vi "initialize_projector.vi"(3 "BlueCurrent":u8=130, 4 "RedBluePatternRepeat":i32=1, 5 "GreenCurrent":u8=135, 6 "Green Only":bool, 7 "RedCurrent":u8=104, 8 "error in":errorcluster, 9 "blue exp_time_us":i32=8215, 10 "red exp_time_us":i32=8215, 11 "green exp_time_us":i32=235) -> (0 "error out":errorcluster)   [LabVIEW 2019]
panel:
  out "numLutEntries":i32
  out "Sequence Validation Results":bool[](array[boolean])
  # "Exposure/Period out of range"
  # "Pattern Number out of range"
  # "continuous TriggerOut1 request or overlapping black sectors"
  # "post vector was not inserted prior to external triggered vector"
  # "frame period or exposure difference is less than 230usec"
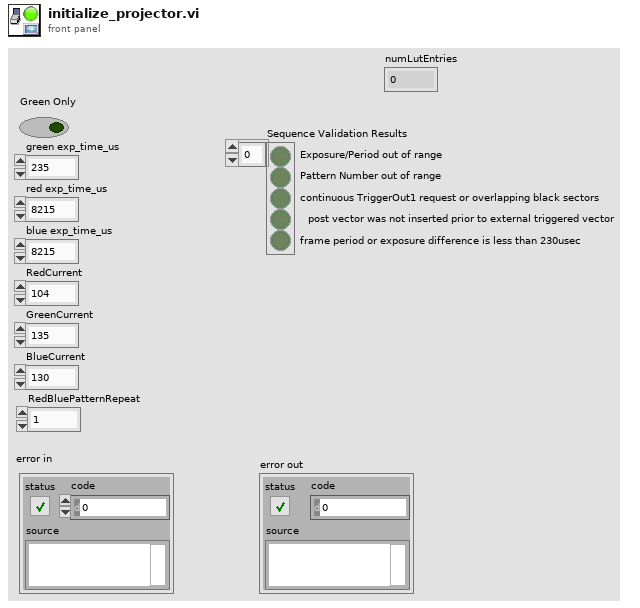
[diagram p1: front panel]
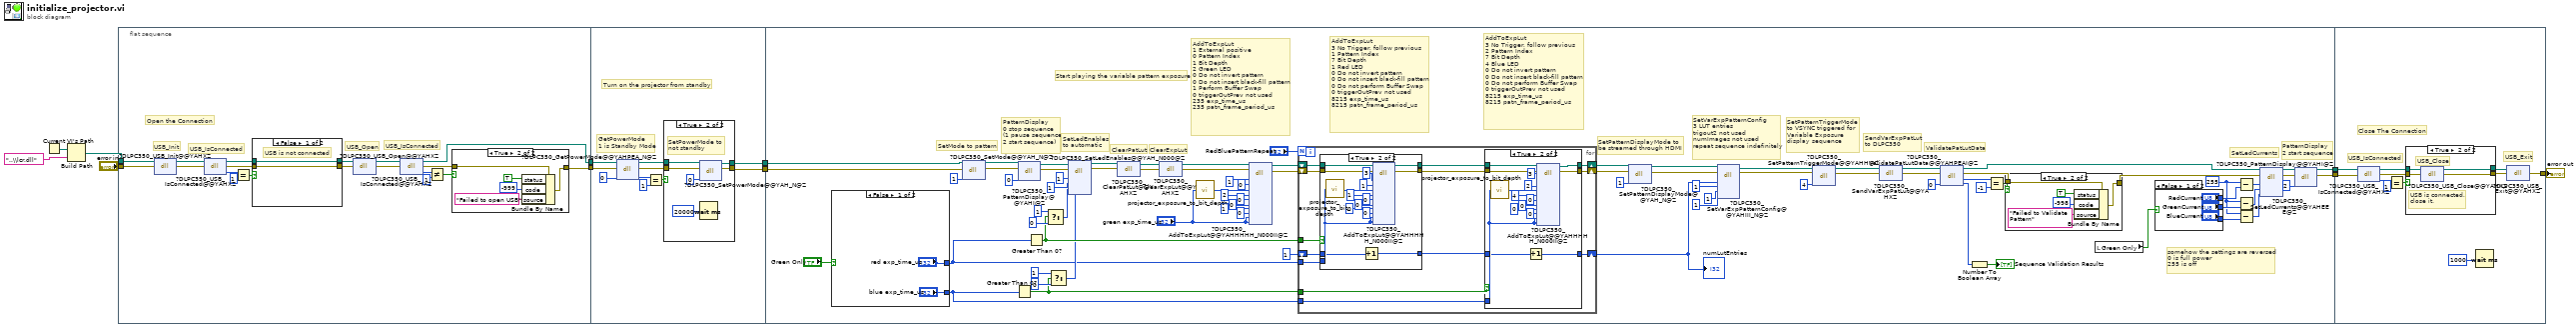
[diagram p0: block diagram]
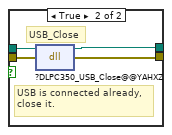
[diagram p3: hidden frame]
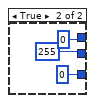
[diagram p7: hidden frame]
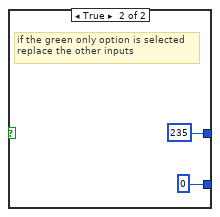
[diagram p8: hidden frame]
diagram:
  n1 = Current VI's Path() -> (path=w6:path)
  n2 = Build Path(base path=w6, name or relative path="..\\lcr.dll") -> (appended path=w4:path)
  n3 = flat-sequence {
    tunnel: [w20] -> w9
    tunnel: "error in" -> [w19]
    tunnel: w4 -> [w18]
    tunnel: [w13] -> w3
    tunnel: w9 -> [w50]
    tunnel: [w52] -> w8
    tunnel: w3 -> [w45]
    tunnel: [w43] -> w2
    tunnel: [w94] -> w10
    tunnel: w8 -> [w108]
    tunnel: w2 -> [w107]
    tunnel: [w92] -> w1
    tunnel: [w209] -> w11
    tunnel: w10 -> [w208]
    tunnel: w1 -> [w207]
    frame #0 {
      # "Open the Connection"
      # "USB_IsConnected"
      # "USB_Open"
      # "USB_IsConnected"
      # "USB_Init"
      n4 = dll-call lib="C:/Users/mochil/Dropbox/LeiferShaevitz/Github/ProjectAPI/LabviewVIs/lcr.dll" fn="?DLPC350_USB_Init@@YAHXZ"(path in=w18, error in=w19) -> (path out=w17:path, error out=w30:errorcluster)  [unwired: 2 in]
      n5 = dll-call lib="C:/Users/mochil/Dropbox/LeiferShaevitz/Github/ProjectAPI/LabviewVIs/lcr.dll" fn="?DLPC350_USB_IsConnected@@YAHXZ"(path in=w17, error in=w30) -> (path out=w16:path, error out=w27:errorcluster, "return type"=w22:i32)  [unwired: 1 in]
      n6 = Equal?(x=w22, y=1) -> (x = y?=w28:bool)
      n7 = case shown="False" w28 {
        tunnel: w27 -> [w38 w42]
        tunnel: [w38 w41] -> w29
        tunnel: w16 -> [w37 w40]
        tunnel: [w37 w39] -> w15
        frame False {
          # "USB is not connected"
        }
        frame True {
          # "USB_Close"
          # "USB is connected already,\nclose it."
          n8 = dll-call lib="C:/Users/mochil/Dropbox/LeiferShaevitz/Github/ProjectAPI/LabviewVIs/lcr.dll" fn="?DLPC350_USB_Close@@YAHXZ"(path in=w40, error in=w42) -> (path out=w39:path, error out=w41:errorcluster)  [unwired: 2 in]
        }
      }
      n9 = dll-call lib="C:/Users/mochil/Dropbox/LeiferShaevitz/Github/ProjectAPI/LabviewVIs/lcr.dll" fn="?DLPC350_USB_Open@@YAHXZ"(path in=w15, error in=w29) -> (path out=w14:path, error out=w26:errorcluster)  [unwired: 2 in]
      n10 = dll-call lib="C:/Users/mochil/Dropbox/LeiferShaevitz/Github/ProjectAPI/LabviewVIs/lcr.dll" fn="?DLPC350_USB_IsConnected@@YAHXZ"(path in=w14, error in=w26) -> (path out=w13:path, error out=w23:errorcluster, "return type"=w12:i32)  [unwired: 1 in]
      n11 = Not Equal?(x=w12, y=1) -> (x != y?=w24:bool)
      n12 = case shown="True" w24 {
        tunnel: w23 -> [w31 w33]
        tunnel: [w31 w32] -> w20
        frame False {
        }
        frame True {
          n13 = Bundle By Name(cluster=w33, "status"=TRUE, "code"=-999, "source"="Failed to open USB") -> (w32:errorcluster)
        }
      }
    }
    frame #1 {
      # "Turn on the projector from standby"
      # "GetPowerMode\n1 is Standby Mode"
      n14 = dll-call lib="C:/Users/mochil/Dropbox/LeiferShaevitz/Github/ProjectAPI/LabviewVIs/lcr.dll" fn="?DLPC350_GetPowerMode@@YAHPEA_N@Z"(path in=w45, error in=w50, "pStandby"=0) -> (path out=w44:path, error out=w46:errorcluster, "pStandby"=w49:i32)  [unwired: 2 in]
      n15 = Equal?(x=w49, y=1) -> (x = y?=w47:bool)
      n16 = case shown="True" w47 {
        tunnel: [w54 w59] -> w52
        tunnel: w46 -> [w54 w58]
        tunnel: w44 -> [w53 w56]
        tunnel: [w53 w55] -> w43
        frame False {
        }
        frame True {
          # "SetPowerMode to\nnot standby"
          n17 = dll-call lib="C:/Users/mochil/Dropbox/LeiferShaevitz/Github/ProjectAPI/LabviewVIs/lcr.dll" fn="?DLPC350_SetPowerMode@@YAH_N@Z"(path in=w56, error in=w58, "Standby"=0) -> (path out=w55:path, error out=w59:errorcluster)  [unwired: 3 in]
          n18 = Wait (ms)(milliseconds to wait=20000) -> ()  [unwired: 1 out]
        }
      }
    }
    frame #2 {
      w87 = u8 255 ("RedCurrent")
      # "ClearExpLut"
      # "somehow the settings are reversed\n0 is full power\n255 is off"
      # "PatternDisplay\n2 start sequence"
      # "SetLedCurrents"
      # "Start playing the variable pattern exposure"
      # "ValidatePatLutData"
      # "SetPatternTriggerMode\nto VSYNC triggered for \nVariable Exposure \ndisplay sequence"
      # "SetPatternDisplayMode to\nbe streamed through HDMI"
      # "AddToExpLut\n3 No Trigger, follow previous\n2 Pattern Index\n7 Bit Depth\n4 Blue LED\n0 Do not invert pattern\n0 Do not insert black-fill pattern\n0 Do not perform Buffer Swap\n0 triggerOutPrev not used\n8215 exp_time_us\n8215 patn_frame_period_us"
      # "AddToExpLut\n3 No Trigger, follow previous\n1 Pattern Index\n7 Bit Depth\n1 Red LED\n0 Do not invert pattern\n0 Do not insert black-fill pattern\n0 Do not perform Buffer Swap\n0 triggerOutPrev not used\n8215 exp_time_us\n8215 patn_frame_period_us"
      # "AddToExpLut\n1 External positive\n0 Pattern Index\n1 Bit Depth\n2 Green LED\n0 Do not invert pattern\n0 Do not insert black-fill pattern\n1 Perform Buffer Swap\n0 triggerOutPrev not used\n235 exp_time_us\n235 patn_frame_period_us"
      # "SendVarExpPatLut\nto DLPC350"
      # "SetVarExpPatternConfig\n3 LUT entries\ntrigout2 not used\nnumImages not used\nrepeat sequence indefinitely"
      # "ClearPatLut"
      # "PatternDisplay\n0 stop sequence\n(1 pause sequence\n2 start sequence)"
      # "SetLedEnables \nto automatic"
      # "SetMode to pattern"
      n19 = case shown="False" "Green Only" {
        tunnel: ["blue exp_time_us" 0 ("blue exp_time_us")] -> w67
        tunnel: ["red exp_time_us" 235 ("red exp_time_us")] -> w66
        frame False {
        }
        frame True {
          # "if the green only option is selected\nreplace the other inputs"
        }
      }
      n20 = dll-call lib="C:/Users/mochil/Dropbox/LeiferShaevitz/Github/ProjectAPI/LabviewVIs/lcr.dll" fn="?DLPC350_SetMode@@YAH_N@Z"(path in=w107, error in=w108, "SLmode"=1) -> (path out=w106:path, error out=w135:errorcluster)  [unwired: 3 in]
      n21 = Greater Than 0?(x=w67) -> (x > 0?=w72:bool)
      n22 = dll-call lib="C:/Users/mochil/Dropbox/LeiferShaevitz/Github/ProjectAPI/LabviewVIs/lcr.dll" fn="?DLPC350_PatternDisplay@@YAHI@Z"(path in=w106, error in=w135, "Action"=0) -> (path out=w105:path, error out=w134:errorcluster)  [unwired: 3 in]
      n23 = Greater Than 0?(x=w66) -> (x > 0?=w77:bool)
      n24 = Select(t=1 ("green"), s=w77, f=0) -> (s? t:f=w76:i32)
      n25 = Select(t=1 ("green"), s=w72, f=0) -> (s? t:f=w73:i32)
      n26 = dll-call lib="C:/Users/mochil/Dropbox/LeiferShaevitz/Github/ProjectAPI/LabviewVIs/lcr.dll" fn="?DLPC350_SetLedEnables@@YAH_N000@Z"(path in=w105, error in=w134, "seqCtrl"=1, "red"=w76, "green"=1, "blue"=w73) -> (path out=w104:path, error out=w133:errorcluster)  [unwired: 6 in]
      n27 = dll-call lib="C:/Users/mochil/Dropbox/LeiferShaevitz/Github/ProjectAPI/LabviewVIs/lcr.dll" fn="?DLPC350_ClearPatLut@@YAHXZ"(path in=w104, error in=w133) -> (path out=w70:path, error out=w71:errorcluster)  [unwired: 2 in]
      n28 = dll-call lib="C:/github/ProjectAPI/LabviewVIs/lcr.dll" fn="?DLPC350_ClearExpLut@@YAHXZ"(path in=w70, error in=w71) -> (path out=w69:path, error out=w68:errorcluster)  [unwired: 2 in]
      n29 = call "projector_exposure_to_bit_depth.vi"("exp_time_us"="green exp_time_us") -> ("BitDepth"=w83:i32)
      n30 = dll-call lib="C:/Users/mochil/Dropbox/LeiferShaevitz/Github/ProjectAPI/LabviewVIs/lcr.dll" fn="?DLPC350_AddToExpLut@@YAHHHHH_N000II@Z"(path in=w69, error in=w68, "TrigType"=1, "PatNum"=0, "BitDepth"=w83, "LEDSelect"=2, "InvertPat"=0, "InsertBlack"=0, "BufSwap"=1, "trigOutPrev"=0, "exp_time_us"="green exp_time_us", "ptn_frame_period_us"="green exp_time_us") -> (path out=w82:path, error out=w81:errorcluster)  [unwired: 12 in]
      n31 = for {
        N: "RedBluePatternRepeat" -> [_]
        tunnel: w77 -> [w144]
        tunnel: w72 -> [w143]
        tunnel: w67 -> [w142]
        tunnel: w66 -> [w141]
        shift-right: [w151] -> w103
        shift-left: w82 -> [w146]
        shift-right: [w139] -> w121
        shift-left: w81 -> [w145]
        shift-right: [w140] -> w62
        shift-left: 1 ("numLutEntries") -> [w150]
        n32 = case shown="True" w144 {
          tunnel: w145 -> [w153 w163]
          tunnel: [w153 w162] -> w148
          tunnel: w146 -> [w154 w161]
          tunnel: [w154 w160] -> w147
          tunnel: w141 -> [_ w159]
          tunnel: w150 -> [w152 w156]
          tunnel: [w152 w157] -> w149
          frame False {
          }
          frame True {
            n33 = call "projector_exposure_to_bit_depth.vi"("exp_time_us"=w159) -> ("BitDepth"=w158:i32)
            n34 = Increment(x=w156) -> (x+1=w157:i32)
            n35 = dll-call lib="C:/Users/mochil/Dropbox/LeiferShaevitz/Github/ProjectAPI/LabviewVIs/lcr.dll" fn="?DLPC350_AddToExpLut@@YAHHHHH_N000II@Z"(path in=w161, error in=w163, "TrigType"=3, "PatNum"=1, "BitDepth"=w158, "LEDSelect"=1, "InvertPat"=0, "InsertBlack"=0, "BufSwap"=0, "trigOutPrev"=0, "exp_time_us"=w159, "ptn_frame_period_us"=w159) -> (path out=w160:path, error out=w162:errorcluster)  [unwired: 12 in]
          }
        }
        n36 = case shown="True" w143 {
          tunnel: w148 -> [w171 w181]
          tunnel: [w171 w180] -> w139
          tunnel: w147 -> [w172 w179]
          tunnel: [w172 w178] -> w151
          tunnel: w142 -> [_ w177]
          tunnel: w149 -> [w170 w174]
          tunnel: [w170 w175] -> w140
          frame False {
          }
          frame True {
            n37 = call "projector_exposure_to_bit_depth.vi"("exp_time_us"=w177) -> ("BitDepth"=w176:i32)
            n38 = Increment(x=w174) -> (x+1=w175:i32)
            n39 = dll-call lib="C:/Users/mochil/Dropbox/LeiferShaevitz/Github/ProjectAPI/LabviewVIs/lcr.dll" fn="?DLPC350_AddToExpLut@@YAHHHHH_N000II@Z"(path in=w179, error in=w181, "TrigType"=3, "PatNum"=2, "BitDepth"=w176, "LEDSelect"=4, "InvertPat"=0, "InsertBlack"=0, "BufSwap"=0, "trigOutPrev"=0, "exp_time_us"=w177, "ptn_frame_period_us"=w177) -> (path out=w178:path, error out=w180:errorcluster)  [unwired: 12 in]
          }
        }
      }
      "numLutEntries" <- w62
      n40 = dll-call lib="C:/Users/mochil/Dropbox/LeiferShaevitz/Github/ProjectAPI/LabviewVIs/lcr.dll" fn="?DLPC350_SetPatternDisplayMode@@YAH_N@Z"(path in=w103, error in=w121, "external"=1) -> (path out=w102:path, error out=w120:errorcluster)  [unwired: 3 in]
      n41 = dll-call lib="C:/Users/mochil/Dropbox/LeiferShaevitz/Github/ProjectAPI/LabviewVIs/lcr.dll" fn="?DLPC350_SetVarExpPatternConfig@@YAHIII_N@Z"(path in=w102, error in=w120, "numLutEntries"=w62, "numPatsForTrigOut2"=1 ("repeat"), "numImages"=1 ("numPatsForTrigOut2"), "repeat"=1 ("numImages")) -> (path out=w101:path, error out=w118:errorcluster)  [unwired: 6 in]
      n42 = dll-call lib="C:/Users/mochil/Dropbox/LeiferShaevitz/Github/ProjectAPI/LabviewVIs/lcr.dll" fn="?DLPC350_SetPatternTriggerMode@@YAHH@Z"(path in=w101, error in=w118, "trigMode"=4) -> (path out=w100:path, error out=w117:errorcluster)  [unwired: 3 in]
      n43 = dll-call lib="C:/Users/mochil/Dropbox/LeiferShaevitz/Github/ProjectAPI/LabviewVIs/lcr.dll" fn="?DLPC350_SendVarExpPatLut@@YAHXZ"(path in=w100, error in=w117) -> (path out=w99:path, error out=w116:errorcluster)  [unwired: 2 in]
      n44 = dll-call lib="C:/Users/mochil/Dropbox/LeiferShaevitz/Github/ProjectAPI/LabviewVIs/lcr.dll" fn="?DLPC350_ValidatePatLutData@@YAHPEAI@Z"(path in=w99, error in=w116, "pStatus"=0) -> (path out=w97:path, error out=w109:errorcluster, "return type"=w112:i32, "pStatus"=w114:i32)  [unwired: 1 in]
      n45 = Number To Boolean Array(number=w114) -> (Boolean array=→"Sequence Validation Results":bool[])
      n46 = Equal?(x=w112, y=-1) -> (x = y?=w110:bool)
      n47 = case shown="True" w110 {
        tunnel: w109 -> [w198 w200]
        tunnel: [w198 w199] -> w96
        frame False {
        }
        frame True {
          n48 = Bundle By Name(cluster=w200, "status"=TRUE, "code"=-998, "source"="Failed to Validate Pattern") -> (w199:errorcluster)
        }
      }
      n49 = local read "Green Only"() -> (w64:bool)
      n50 = case shown="False" w64 {
        tunnel: ["RedCurrent" u8 0 ("RedCurrent")] -> w90
        tunnel: ["GreenCurrent" u8 255 ("GreenCurrent")] -> w89
        tunnel: ["BlueCurrent" u8 0 ("BlueCurrent")] -> w86
        frame False {
        }
        frame True {
        }
      }
      n51 = Subtract(x=w87, y=w90) -> (x-y=w91:u8)
      n52 = Subtract(x=w87, y=w89) -> (x-y=w88:u8)
      n53 = Subtract(x=w87, y=w86) -> (x-y=w85:u8)
      n54 = dll-call lib="C:/Users/mochil/Dropbox/LeiferShaevitz/Github/ProjectAPI/LabviewVIs/lcr.dll" fn="?DLPC350_SetLedCurrents@@YAHEEE@Z"(path in=w97, error in=w96, "RedCurrent"=w91, "GreenCurrent"=w88, "BlueCurrent"=w85) -> (path out=w93:path, error out=w95:errorcluster)  [unwired: 5 in]
      n55 = dll-call lib="C:/Users/mochil/Dropbox/LeiferShaevitz/Github/ProjectAPI/LabviewVIs/lcr.dll" fn="?DLPC350_PatternDisplay@@YAHI@Z"(path in=w93, error in=w95, "Action"=2) -> (path out=w92:path, error out=w94:errorcluster)  [unwired: 3 in]
    }
    frame #3 {
      # "Close The Connection"
      # "USB_Exit"
      # "USB_IsConnected"
      n56 = dll-call lib="C:/Users/mochil/Dropbox/LeiferShaevitz/Github/ProjectAPI/LabviewVIs/lcr.dll" fn="?DLPC350_USB_IsConnected@@YAHXZ"(path in=w207, error in=w208) -> (path out=w206:path, error out=w212:errorcluster, "return type"=w213:i32)  [unwired: 1 in]
      n57 = Equal?(x=w213, y=1) -> (x = y?=w211:bool)
      n58 = case shown="True" w211 {
        tunnel: w212 -> [w216 w220]
        tunnel: [w216 w219] -> w214
        tunnel: w206 -> [w215 w218]
        tunnel: [w215 w217] -> w205
        frame False {
          # "USB is not connected"
        }
        frame True {
          # "USB_Close"
          # "USB is connected,\nclose it."
          n59 = dll-call lib="C:/Users/mochil/Dropbox/LeiferShaevitz/Github/ProjectAPI/LabviewVIs/lcr.dll" fn="?DLPC350_USB_Close@@YAHXZ"(path in=w218, error in=w220) -> (path out=w217:path, error out=w219:errorcluster)  [unwired: 2 in]
        }
      }
      n60 = Wait (ms)(milliseconds to wait=1000) -> ()  [unwired: 1 out]
      n61 = dll-call lib="C:/Users/mochil/Dropbox/LeiferShaevitz/Github/ProjectAPI/LabviewVIs/lcr.dll" fn="?DLPC350_USB_Exit@@YAHXZ"(path in=w205, error in=w214) -> (error out=w209:errorcluster)  [unwired: 2 in, 1 out]
    }
  }
  "error out" <- w11
